vi "test rotate picture.3.vi"() -> ()   [LabVIEW 2020]
uses:
  <vilib>/picture/picture.llb/imagedata.ctl
panel:
  in  "Zoom to fit":bool caption="Actual size"
  out "24-bit pixmap 2":u32[][](array[numeric]) format="%x"
  out "image data 2":T1
  out "24-bit pixmap":u32[][](array[numeric]) format="%x"
  in  "Clockwise":bool caption="CounterClockwise"
  out "image data":T1
  out "image":u8[](array[numeric])
  out "Picture 2":picture
  out "Picture":picture
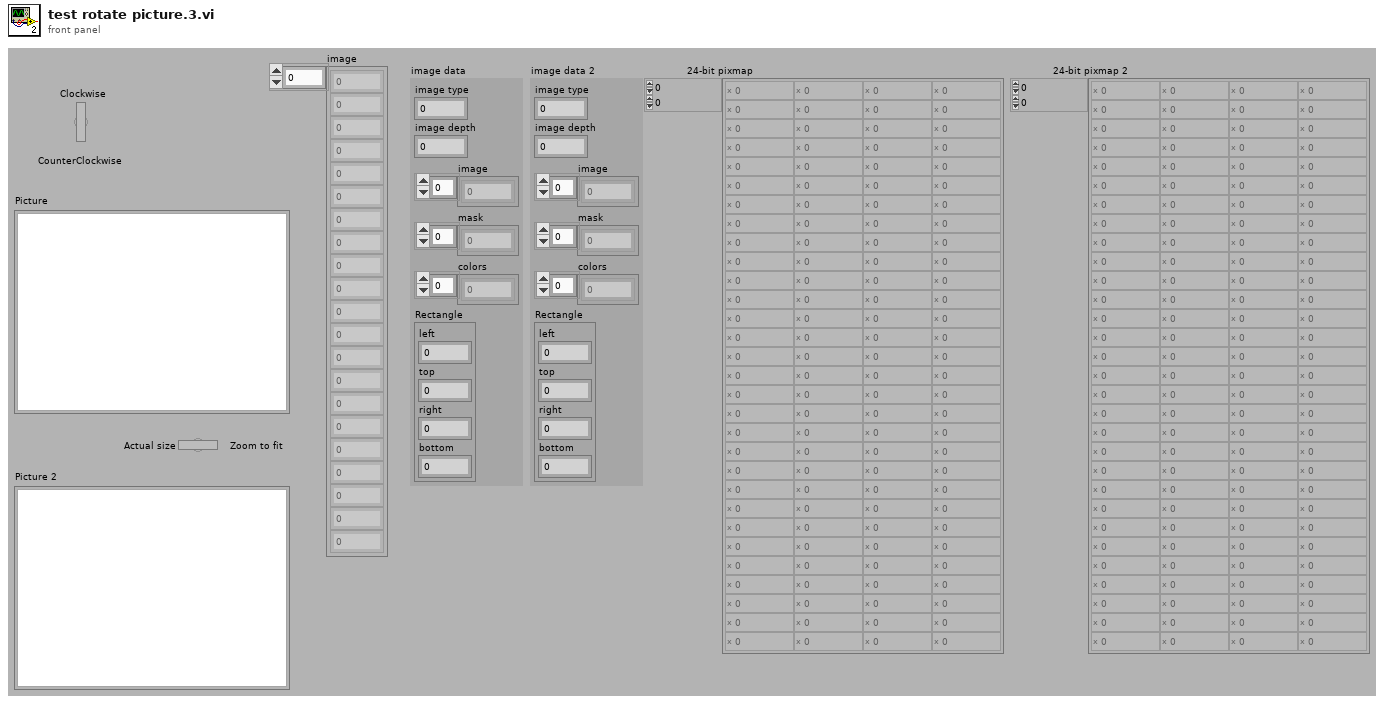
[diagram p1: front panel]
types:
  T1 = typedef "imagedata.ctl" = cluster{"image type":i32, "image depth":i32, "image":u8[], "mask":u8[], "colors":u32[], "Rectangle":cluster{"left":i16, "top":i16, "right":i16, "bottom":i16}}
  T2 = cluster{"left":i16, "top":i16, "right":i16, "bottom":i16}
  T3 = typedef "LVBoundsTypeDef.ctl" = cluster{"Width":u32, "Height":u32}
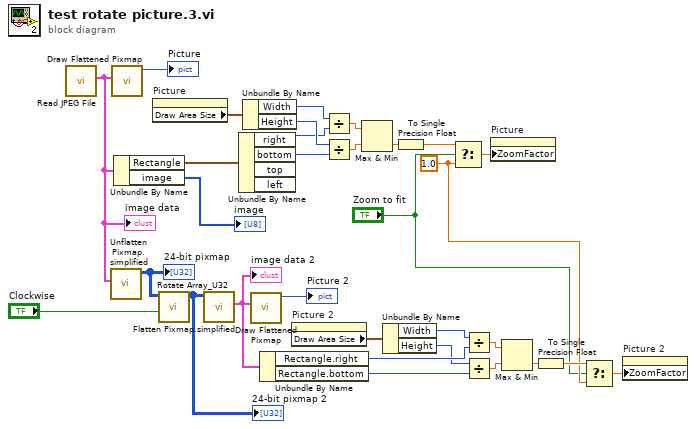
[diagram p0: block diagram]
diagram:
  w2 = sgl 1.0 ("f")
  n1 = call <vilib>:"Read JPEG File.vi"() -> ("image data"=w19:T1)  [unwired: 9 in, 2 out]
  "image data" <- w19
  n2 = call "Unflatten Pixmap.simplified.vi"("image data"=w19) -> ("24-bit pixmap"=w17:u32[][])  [unwired: 10 in]
  "24-bit pixmap" <- w17
  n3 = call <vilib>:"Draw Flattened Pixmap.vi"("image data"=w19) -> ("new picture"=→"Picture":picture)  [unwired: 8 in]
  n4 = Unbundle By Name(w19) -> ("Rectangle"=w24:T2, "image"=→"image":u8[])
  n5 = property on="Picture" class="Pict"() -> ("Draw Area Size"=w30:T3)  [unwired: 2 in, 2 out]
  n6 = call "Rotate Array_U32.vi"("Clockwise"="Clockwise", "Array"=w17) -> ("Rotated Array"=w7:u32[][])  [unwired: 9 in]
  "24-bit pixmap 2" <- w7
  n7 = call "Flatten Pixmap.simplified.vi"("24-bit pixmap"=w7) -> ("image data"=w16:T1)  [unwired: 10 in]
  "image data 2" <- w16
  n8 = Unbundle By Name(w24) -> ("right"=w21:i16, "bottom"=w20:i16)  [unwired: 2 out]
  n9 = Unbundle By Name(w30) -> ("Width"=w26:u32, "Height"=w27:u32)
  n10 = call <vilib>:"Draw Flattened Pixmap.vi"("image data"=w16) -> ("new picture"=→"Picture 2":picture)  [unwired: 8 in]
  n11 = Unbundle By Name(w16) -> ("Rectangle.right"=w10:i16, "Rectangle.bottom"=w8:i16)
  n12 = property on="Picture 2" class="Pict"() -> ("Draw Area Size"=w12:T3)  [unwired: 2 in, 2 out]
  n13 = Divide(x=w26, y=w21) -> (x/y=w28:dbl)
  n14 = Divide(x=w27, y=w20) -> (x/y=w29:dbl)
  n15 = Max & Min(x=w28, y=w29) -> (min(x,y)=w25:dbl)  [unwired: 1 out]
  n16 = Unbundle By Name(w12) -> ("Width"=w11:u32, "Height"=w9:u32)
  n17 = To Single Precision Float(number=w25) -> (single precision float=w3:sgl)
  n18 = Select(t=w3, s="Zoom to fit", f=w2) -> (s? t:f=w4:sgl)
  n19 = Divide(x=w11, y=w10) -> (x/y=w14:dbl)
  n20 = Divide(x=w9, y=w8) -> (x/y=w13:dbl)
  n21 = property on="Picture" class="Pict"("ZoomFactor"=w4) -> ()  [unwired: 2 in, 2 out]
  n22 = Max & Min(x=w14, y=w13) -> (min(x,y)=w15:dbl)  [unwired: 1 out]
  n23 = To Single Precision Float(number=w15) -> (single precision float=w6:sgl)
  n24 = Select(t=w6, s="Zoom to fit", f=w2) -> (s? t:f=w5:sgl)
  n25 = property on="Picture 2" class="Pict"("ZoomFactor"=w5) -> ()  [unwired: 2 in, 2 out]
